vi "OA_Controller_L.vi"(9 "Gait Phase":dbl, 10 "Weight":dbl, 11 "Walking Speed":dbl) -> (3 "Torque Output":dbl)   [LabVIEW 2019]
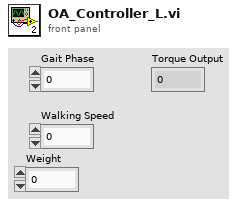
[diagram p1: front panel]
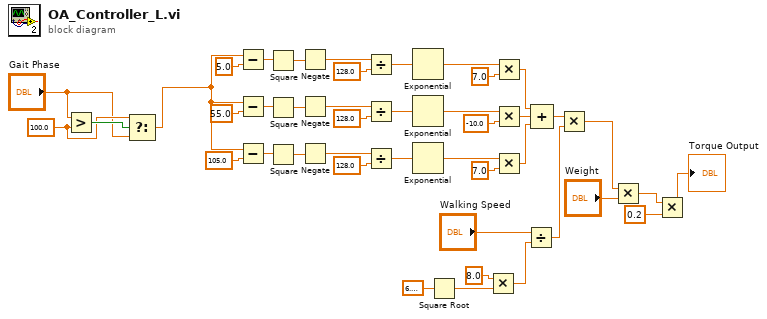
[diagram p0: block diagram]
diagram:
  w3 = 100.0 ("y")
  n1 = Greater?(x="Gait Phase", y=w3) -> (0:w4:bool)
  n2 = Select(t=w3, s=w4, f="Gait Phase") -> (s? t:f=w1:dbl)
  n3 = Subtract(x=w1, y=5.0) -> (x-y=w10:dbl)
  n4 = Subtract(x=w1, y=55.0) -> (x-y=w18:dbl)
  n5 = Subtract(x=w1, y=105.0) -> (x-y=w26:dbl)
  n6 = Square(x=w10) -> (x^2=w11:dbl)
  n7 = Square(x=w18) -> (x^2=w19:dbl)
  n8 = Square(x=w26) -> (x^2=w27:dbl)
  n9 = Negate(x=w11) -> (-x=w12:dbl)
  n10 = Negate(x=w19) -> (-x=w20:dbl)
  n11 = Negate(x=w27) -> (-x=w28:dbl)
  n12 = Divide(x=w12, y=128.0) -> (x/y=w14:dbl)
  n13 = Divide(x=w20, y=128.0) -> (x/y=w22:dbl)
  n14 = Divide(x=w28, y=128.0) -> (x/y=w30:dbl)
  n15 = Exponential(1:w14) -> (0:w15:dbl)
  n16 = Exponential(1:w22) -> (0:w23:dbl)
  n17 = Exponential(1:w30) -> (0:w31:dbl)
  n18 = Square Root(x=6.283185307179586) -> (sqrt(x)=w42:dbl)
  n19 = Multiply(x=8.0, y=w42) -> (x*y=w40:dbl)
  n20 = Multiply(x=w15, y=7.0) -> (x*y=w34:dbl)
  n21 = Multiply(x=w23, y=-10.0) -> (x*y=w35:dbl)
  n22 = Multiply(x=w31, y=7.0) -> (x*y=w36:dbl)
  n23 = Divide(x="Walking Speed", y=w40) -> (x/y=w38:dbl)
  n24 = Compound Arithmetic op=ADD(w34, w35, w36) -> (w37:dbl)
  n25 = Multiply(x=w37, y=w38) -> (x*y=w9:dbl)
  n26 = Multiply(x=w9, y="Weight") -> (x*y=w7:dbl)
  n27 = Multiply(x=w7, y=0.2) -> (x*y=→"Torque Output":dbl)
